vi "Read Scope Channel.vi"(8 "error in (no error)":errorcluster, 11 "Scope Channel configuration":refnum<class "Scope Channel configuration.lvclass">) -> (0 "error out":errorcluster, 2 "Scope Channel Setting":T1={"Gain"=1, "Offset"=0, "Vertical Range"=10.0, "Vertical Offset"=0.0, "Unit"="V", "Attenuation"=1.0, "Vertical Coupling"="DC", "Impedance"="1M", "Auto Setup"=TRUE}, 3 "Scope Channel configuration out":refnum<class "Scope Channel configuration.lvclass">)   [LabVIEW 2025, in "Scope.lvlib" / "Scope Channel configuration.lvclass"]
uses:
  Scope Channel configuration.lvclass
  Scope Channel Setting.ctl
  Scope Channel configuration.lvclass/Scope Channel configuration.ctl
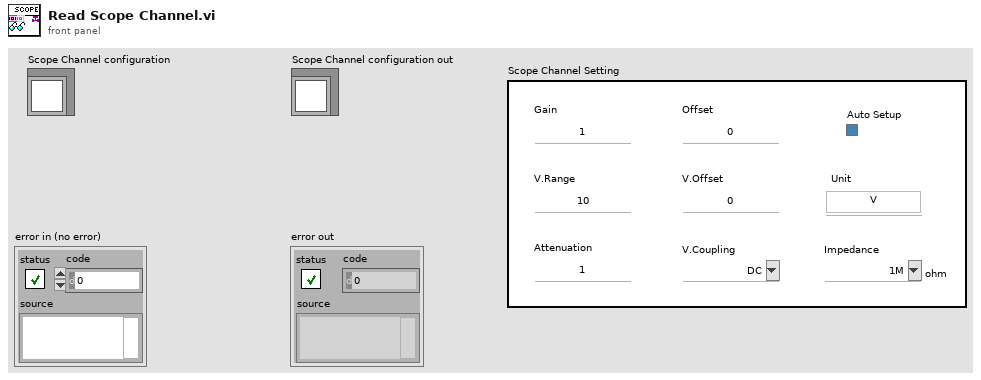
[diagram p1: front panel]
types:
  T1 = typedef "Scope.lvlib/Scope Channel configuration.lvclass/Scope Channel Setting.ctl" = cluster{"Gain":u32, "Offset":u32, "Vertical Range":dbl, "Vertical Offset":dbl, "Unit":string, "Attenuation":dbl, "Vertical Coupling":string, "Impedance":string, "Auto Setup":bool}
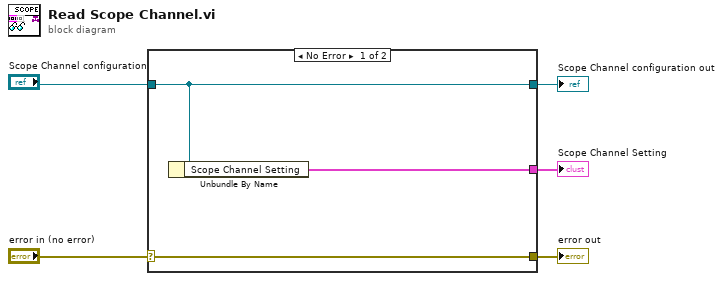
[diagram p0: block diagram]
diagram:
  n1 = case shown="No Error" "error in (no error)" {
    selector: "error in (no error)" -> [w8 w9]
    tunnel: [w8 w9] -> w4
    tunnel: [w7 w10] -> w2
    tunnel: "Scope Channel configuration" -> [w7 w10]
    tunnel: [w6 _] -> w1
    frame No Error {
      n2 = Unbundle By Name(w7) -> ("Scope Channel Setting"=w6:T1)
    }
    frame Error {
    }
  }
  "error out" <- w4
  "Scope Channel configuration out" <- w2
  "Scope Channel Setting" <- w1
